vi "Status Preset.vi"(8 "error in":errorcluster, 11 "Instrument Handle In":i32) -> (0 "error out":errorcluster, 3 "Instrument Handle Out":i32)   [LabVIEW 8.6, in "ZTScopeM.lvlib"]
doc: "Sets the status reporting event enable data structures to a known state. The condition and event register contents are not affected. All device-dependent status registers which cascade events into the Questionable Status and the Operation Status Registers are enabled by setting those device-dependent event enable registers to 7FFF16 (the 15 LSBs set). The IEEE-488.2 mandatory status data structures are disabled by setting the Questionable Status and Operation Status event enable registers to 000016. The Status Byte and Standard Event Status Registers as defined by IEEE 488.2 are not affected."
uses:
  ZTScopeM.lvlib
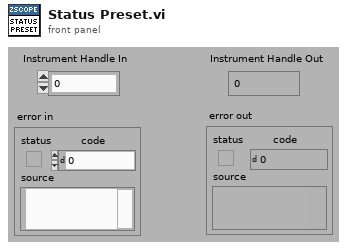
[diagram p1: front panel]
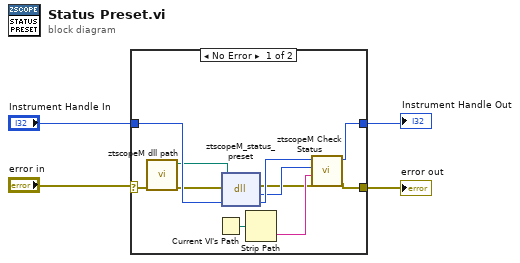
[diagram p0: block diagram]
diagram:
  n1 = case shown="No Error" "error in" {
    selector: "error in" -> [w8 w17]
    tunnel: [w10 w17] -> w1
    tunnel: "Instrument Handle In" -> [w15 w16]
    tunnel: [w9 w16] -> w3
    frame #0 {
      n2 = call "ztscopeM dll path.vi"("error in (no error)"=w8) -> ("error out"=w6:errorcluster, "<instrument>.dll path"=w7:path)  [unwired: 9 in]
      n3 = Current VI's Path() -> (path=w14:path)
      n4 = dll-call lib="C:/Program Files (x86)/National Instruments/LabVIEW 2013/instr.lib/ztscopem/ztscopeM.dll" fn="ztscopeM_status_preset"(path in=w7, error in=w6, "instrument handle"=w15) -> (error out=w5:errorcluster, "status"=w11:i32, "instrument handle"=w12:i32)  [unwired: 1 in, 1 out]
      n5 = Strip Path(path=w14) -> (name=w13:string)  [unwired: 1 out]
      n6 = call "ztscopeM Check Status.vi"("error in"=w5, "name of VI"=w13, "status (return code)"=w11, "instrument handle in"=w12) -> ("error out"=w10:errorcluster, "instrument handle out"=w9:i32)  [unwired: 2 in]
    }
    frame #1 {
    }
  }
  "Instrument Handle Out" <- w3
  "error out" <- w1
